vi "List Sections.vi"(8 "error in (no error)":errorcluster, 11 "Ini Path in":path) -> (0 "error out":errorcluster, 2 "Sections":string[](array[string]), 3 "Ini Path out":path)   [LabVIEW 2018, in "Cfg.lvlib"]
uses:
  Cfg.lvlib
  Action.ctl
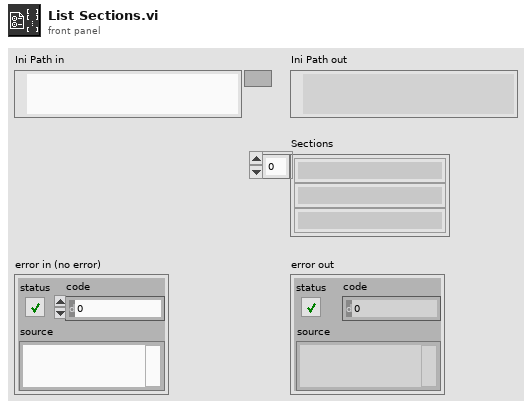
[diagram p1: front panel]
types:
  T1 = typedef "Cfg.lvlib/Action.ctl" = enum8{"noop", "new", "read_or_create", "read", "write", "remove", "keys", "sections", "remove_section", "import", "export", "get", "set", "pop", "add", "list", "list_sections", "pop_section"}
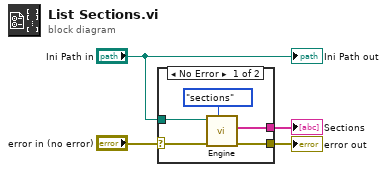
[diagram p0: block diagram]
diagram:
  n1 = case shown="No Error" "error in (no error)" {
    selector: "error in (no error)" -> [w9 w10]
    tunnel: "Ini Path in" -> [w7 _]
    tunnel: [w6 _] -> w2
    tunnel: [w5 w10] -> w1
    frame No Error {
      n2 = call "Engine.vi"("Action"=Action."sections", "error in (no error)"=w9, "INI Path in"=w7) -> ("error out"=w5:errorcluster, "skvc out"=w6:string[])  [unwired: 5 in, 2 out]
    }
    frame Error {
    }
  }
  "error out" <- w1
  "Sections" <- w2
  "Ini Path out" <- "Ini Path in"
